vi "Set Server Address.vi"(10 "Server Address":string, 11 "OOP Server in":refnum<class "Streamer_server.lvclass">) -> (3 "OOP Server out":refnum<class "Streamer_server.lvclass">)   [LabVIEW 2019, in "Streamer_server.lvlib" / "Streamer_server.lvclass"]
uses:
  Streamer_server.lvclass
  Streamer_server.lvclass/Streamer_server.ctl
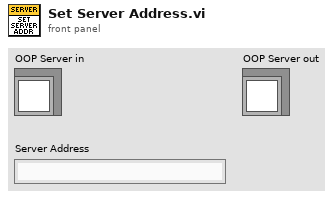
[diagram p1: front panel]
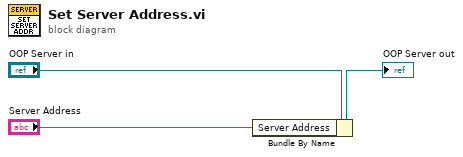
[diagram p0: block diagram]
diagram:
  n1 = Bundle By Name(cluster="OOP Server in", "Server Address"="Server Address") -> (→"OOP Server out":refnum<class "Streamer_server.lvclass">)
